vi "rethinkdb_json_from_cluster.vi"(8 "error in (no error)":errorcluster, 10 "key":string, 11 "cluster":variant) -> (0 "error out":errorcluster, 3 "json":string)   [LabVIEW 2017]
uses:
  <vilib>/Utility/Data Type/NI_Data Type.lvlib
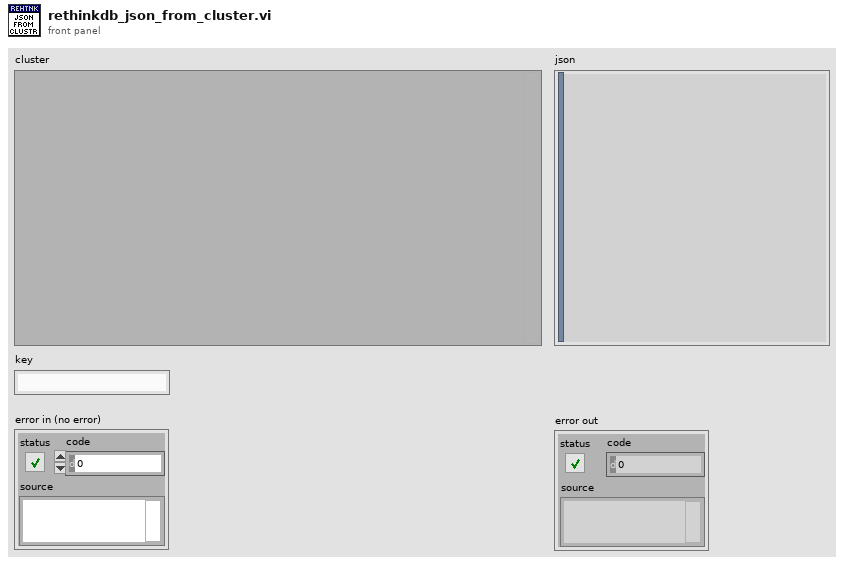
[diagram p1: front panel]
types:
  T1 = typedef "NI_Data Type.lvlib/Data Type.ctl" = enum8{"Invalid Type", "Void", "I8", "I16", "I32", "I64", "U8", "U16", "U32", "U64", "Single Float", "Double Float", "Extended Float", "Single Complex", "Double Complex", "Extended Complex", "Enum U8", "Enum U16", "Enum U32", "Enum U64", "Single Float With Unit", "Double Float With Unit", "Extended Float With Unit", "Single Complex with Unit", "Double Complex with Unit", "Extended Complex with Unit", "Boolean", "String", "Path", "Picture", "Tag", "Array", "Cluster", "Variant", "LV Variant", "Waveform", "Timestamp", "Digital Waveform", "Digital Data", "ExpressData", "Refnum", "External Data", "VI", "Poly VI", "LabVIEW Class Instance", "Fixed Point"}
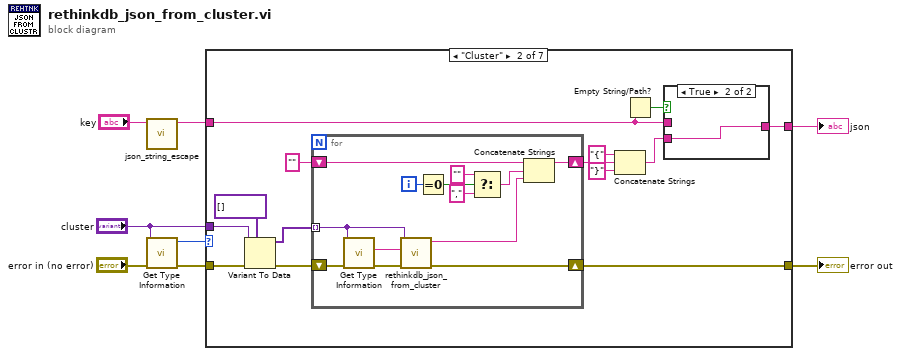
[diagram p0: block diagram]
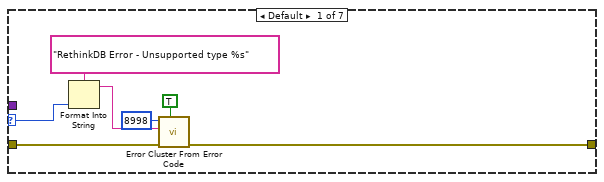
[diagram p2: hidden frame]
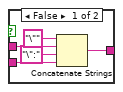
[diagram p3: hidden frame]
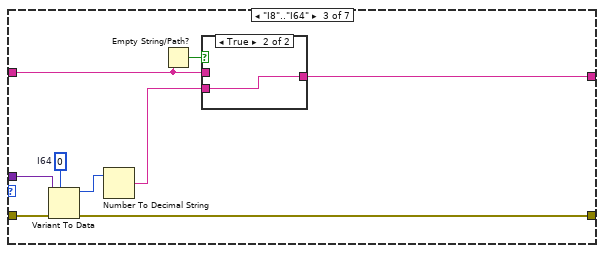
[diagram p4: hidden frame]
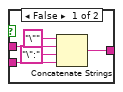
[diagram p5: hidden frame]
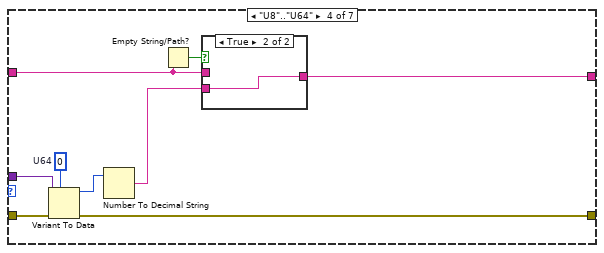
[diagram p6: hidden frame]
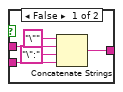
[diagram p7: hidden frame]
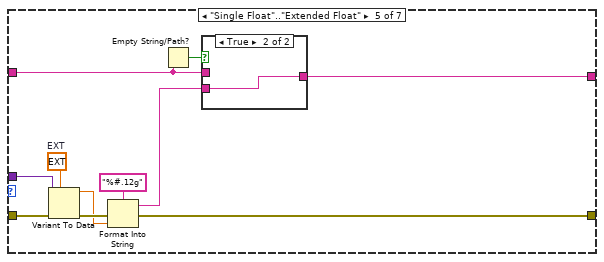
[diagram p8: hidden frame]
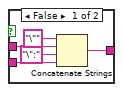
[diagram p9: hidden frame]
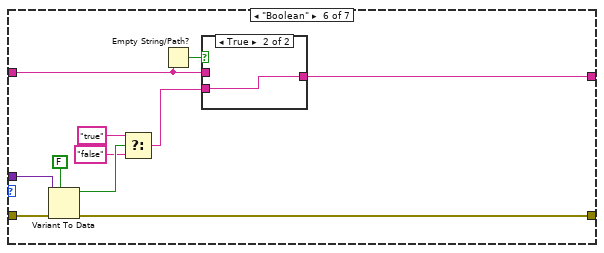
[diagram p10: hidden frame]
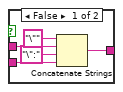
[diagram p11: hidden frame]
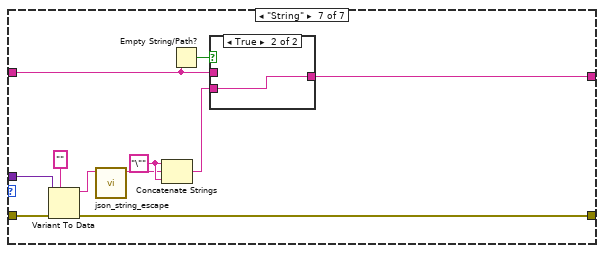
[diagram p12: hidden frame]
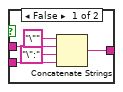
[diagram p13: hidden frame]
diagram:
  n1 = call "json_string_escape.vi"("string"="key") -> ("escaped string"=w1:string)  [unwired: 10 in]
  n2 = call <vilib>:"Get Type Information.vi"("error in (no error)"="error in (no error)", "Variant"="cluster") -> ("error out"=w5:errorcluster, "Type"=w7:T1)  [unwired: 5 in, 3 out]
  n3 = case shown="\"Cluster\"" w7 {
    selector: w7 -> [w11 _ _ _ _ _ _]
    tunnel: "cluster" -> [_ w28 w56 w71 w88 w105 w122]
    tunnel: w5 -> [w15 w29 w57 w72 w89 w106 w123]
    tunnel: [w14 w26 w52 w67 w82 w100 w118] -> w4
    tunnel: [_ w21 w51 w66 w85 w104 w121] -> w3
    tunnel: w1 -> [_ w20 w50 w65 w84 w103 w120]
    frame Default {
      n4 = Format Into String(format string="RethinkDB Error - Unsupported type %s" ("error message (\"\")"), w11) -> (resulting string=w9:string)  [unwired: 2 in, 1 out]
      n5 = call <vilib>:"Error Cluster From Error Code.vi"("show call chain? (False)"=TRUE, "error in (no error)"=w15, "error message (\"\")"=w9, "error code (0)"=8998) -> ("error out"=w14:errorcluster)  [unwired: 5 in]
    }
    frame "Cluster" {
      n6 = Variant To Data(error in=w29, type=variant[] [], Variant=w28) -> (data=w24:variant[], error out=w25:errorcluster)
      n7 = for {
        shift-right: [w48] -> w26
        shift-left: w25 -> [w47]
        tunnel: w24 -> [w45] mode=indexing
        shift-right: [w42] -> w19
        shift-left: "" -> [w43]
        i -> [w41]
        n8 = call <vilib>:"Get Type Information.vi"("error in (no error)"=w47, "Variant"=w45) -> ("error out"=w46:errorcluster, "Name"=w44:string)  [unwired: 5 in, 3 out]
        n9 = call "rethinkdb_json_from_cluster.vi"("error in (no error)"=w46, "key"=w44, "cluster"=w45) -> ("error out"=w48:errorcluster, "json"=w40:string)  [unwired: 7 in]
        n10 = Equal To 0?(x=w41) -> (x = 0?=w39:bool)
        n11 = Select(t="", s=w39, f="," ("string")) -> (s? t:f=w36:string)
        n12 = Concatenate Strings(w43, w36, w40) -> (w42:string)
      }
      n13 = Concatenate Strings("{" ("string"), w19, "}" ("string")) -> (w18:string)
      n14 = Empty String/Path?(string/path=w20) -> (empty?=w22:bool)
      n15 = case shown="True" w22 {
        tunnel: w18 -> [w32 w35]
        tunnel: [w31 w35] -> w21
        tunnel: w20 -> [w30 _]
        frame False {
          n16 = Concatenate Strings("\"" ("string"), w30, "\":" ("string"), w32) -> (w31:string)
        }
        frame True {
        }
      }
    }
    frame "I8".."I64" {
      w55 = i64 0  # I64
      n17 = Variant To Data(error in=w57, type=w55, Variant=w56) -> (data=w54:i64, error out=w52:errorcluster)
      n18 = Number To Decimal String(number=w54) -> (decimal integer string=w53:string)  [unwired: 1 in]
      n19 = Empty String/Path?(string/path=w50) -> (empty?=w49:bool)
      n20 = case shown="True" w49 {
        tunnel: w53 -> [w60 w63]
        tunnel: [w59 w63] -> w51
        tunnel: w50 -> [w58 _]
        frame False {
          n21 = Concatenate Strings("\"" ("string"), w58, "\":" ("string"), w60) -> (w59:string)
        }
        frame True {
        }
      }
    }
    frame "U8".."U64" {
      w70 = u64 0  # U64
      n22 = Variant To Data(error in=w72, type=w70, Variant=w71) -> (data=w69:u64, error out=w67:errorcluster)
      n23 = Number To Decimal String(number=w69) -> (decimal integer string=w68:string)  [unwired: 1 in]
      n24 = Empty String/Path?(string/path=w65) -> (empty?=w64:bool)
      n25 = case shown="True" w64 {
        tunnel: w68 -> [w75 w78]
        tunnel: [w74 w78] -> w66
        tunnel: w65 -> [w73 _]
        frame False {
          n26 = Concatenate Strings("\"" ("string"), w73, "\":" ("string"), w75) -> (w74:string)
        }
        frame True {
        }
      }
    }
    frame "Single Float".."Extended Float" {
      w87 = ext 0.0  # EXT
      n27 = Variant To Data(error in=w89, type=w87, Variant=w88) -> (data=w81:ext, error out=w86:errorcluster)
      n28 = Format Into String(format string="%#.12g", error in=w86, w81) -> (resulting string=w79:string, error out=w82:errorcluster)  [unwired: 1 in]
      n29 = Empty String/Path?(string/path=w84) -> (empty?=w83:bool)
      n30 = case shown="True" w83 {
        tunnel: w79 -> [w92 w95]
        tunnel: [w91 w95] -> w85
        tunnel: w84 -> [w90 _]
        frame False {
          n31 = Concatenate Strings("\"" ("string"), w90, "\":" ("string"), w92) -> (w91:string)
        }
        frame True {
        }
      }
    }
    frame "Boolean" {
      n32 = Variant To Data(error in=w106, type=FALSE, Variant=w105) -> (data=w99:bool, error out=w100:errorcluster)
      n33 = Select(t="true", s=w99, f="false") -> (s? t:f=w98:string)
      n34 = Empty String/Path?(string/path=w103) -> (empty?=w102:bool)
      n35 = case shown="True" w102 {
        tunnel: w98 -> [w109 w112]
        tunnel: [w108 w112] -> w104
        tunnel: w103 -> [w107 _]
        frame False {
          n36 = Concatenate Strings("\"" ("string"), w107, "\":" ("string"), w109) -> (w108:string)
        }
        frame True {
        }
      }
    }
    frame "String" {
      w115 = "\"" ("string")
      n37 = Variant To Data(error in=w123, type="", Variant=w122) -> (data=w114:string, error out=w118:errorcluster)
      n38 = call "json_string_escape.vi"("string"=w114) -> ("escaped string"=w113:string)  [unwired: 10 in]
      n39 = Concatenate Strings(w115, w113, w115) -> (w116:string)
      n40 = Empty String/Path?(string/path=w120) -> (empty?=w119:bool)
      n41 = case shown="True" w119 {
        tunnel: w116 -> [w126 w129]
        tunnel: [w125 w129] -> w121
        tunnel: w120 -> [w124 _]
        frame False {
          n42 = Concatenate Strings("\"" ("string"), w124, "\":" ("string"), w126) -> (w125:string)
        }
        frame True {
        }
      }
    }
  }
  "json" <- w3
  "error out" <- w4
